vi "Ocelot.vi"(9 "RCW (X2)":dbl(slide) scale=-1.0..1.0, 10 "FWD (Y)":dbl(slide) scale=-1.0..1.0, 11 "STR (X)":dbl(slide) scale=-1.0..1.0) -> (0 "FRD":dbl(slide) scale=-1.0..1.0, 1 "FLD":dbl(slide) scale=-1.0..1.0, 2 "BRS":dbl(knob) scale=0.0..360.0, 3 "BLS":dbl(knob) scale=0.0..360.0, 4 "BLD":dbl(slide) scale=-1.0..1.0, 5 "FRS":dbl(knob) scale=0.0..360.0, 6 "BRD":dbl(slide) scale=-1.0..1.0, 7 "FLS":dbl(knob) scale=0.0..360.0)   [LabVIEW 2012]
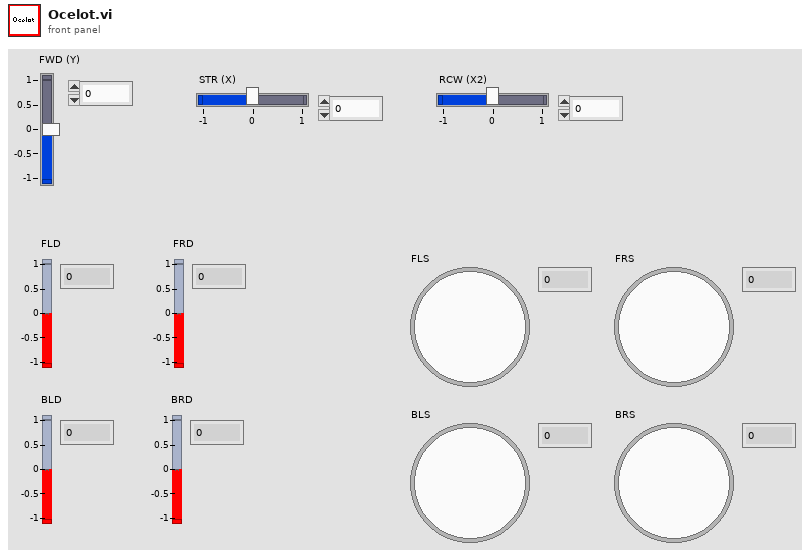
[diagram p1: front panel]
types:
  T1 = cluster{"WD1":dbl, "WD2":dbl, "WD3":dbl, "WD4":dbl}
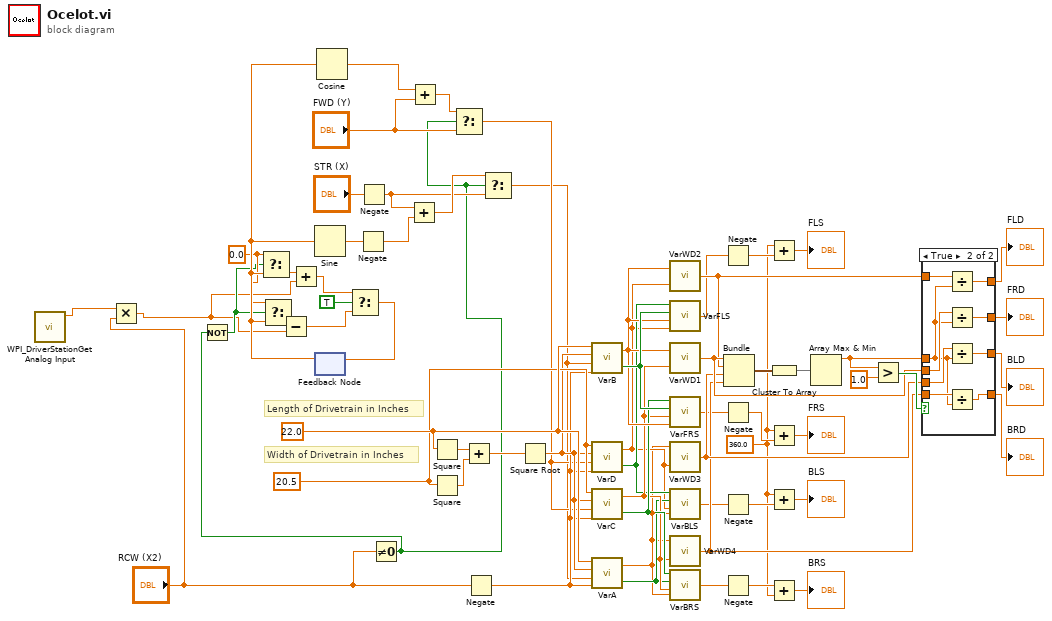
[diagram p0: block diagram]
diagram:
  w6 = 0.0 ("t")
  w32 = 360.0
  w59 = 20.5 ("W")
  w61 = 22.0 ("L")
  # "Length of Drivetrain in Inches"
  # "Width of Drivetrain in Inches"
  n1 = call <vilib>:"WPI_DriverStationGet Analog Input.vi"() -> ("Analog 1 (V)"=w1:dbl)  [unwired: 8 in, 3 out]
  n2 = Multiply(x=w1, y="RCW (X2)") -> (x*y=w2:dbl)
  n3 = feedback #1() -> (w19:dbl)  [unwired: 1 in]
  n4 = Sine(x=w19) -> (sin(x)=w14:dbl)
  n5 = Cosine(x=w19) -> (cos(x)=w18:dbl)
  n6 = Negate(x=w14) -> (-x=w13:dbl)
  n7 = Negate(x="STR (X)") -> (-x=w11:dbl)
  n8 = Not Equal To 0?(x="RCW (X2)") -> (x != 0?=w4:bool)
  n9 = Not(x=w4) -> (.not. x?=w5:bool)
  n10 = Select(t=w6, s=w5, f=w19) -> (s? t:f=w8:dbl)
  n11 = Select(t=w6, s=w5, f=w19) -> (s? t:f=w7:dbl)
  n12 = Subtract(x=w7, y=w2) -> (x-y=w22:dbl)
  n13 = Add(x=w8, y=w2) -> (x+y=w21:dbl)
  n14 = Select(t=w21, s=TRUE, f=w22) -> (s? t:f=w20:dbl)
  n15 = feedback-in #1(w20) -> ()
  n16 = Add(x=w11, y=w13) -> (x+y=w12:dbl)
  n17 = Add(x=w18, y="FWD (Y)") -> (x+y=w17:dbl)
  n18 = Square(x=w61) -> (x^2=w64:dbl)
  n19 = Square(x=w59) -> (x^2=w63:dbl)
  n20 = Select(t=w17, s=w4, f="FWD (Y)") -> (s? t:f=w16:dbl)
  n21 = Add(x=w64, y=w63) -> (x+y=w62:dbl)
  n22 = Negate(x="RCW (X2)") -> (-x=w23:dbl)
  n23 = Select(t=w12, s=w4, f=w11) -> (s? t:f=w10:dbl)
  n24 = Square Root(x=w62) -> (sqrt(x)=w58:dbl)
  n25 = call "VarB.vi"("RCW (X2)"=w23, "STR (X)"=w10, "R"=w58, "L"=w61) -> ("B = 0?"=w48:bool, "B"=w47:dbl)
  n26 = call "VarD.vi"("RCW (X2)"=w23, "FWD (Y)"=w16, "R"=w58, "W"=w59) -> ("x = 0?"=w44:bool, "D"=w42:dbl)
  n27 = call "VarC.vi"("RCW (X2)"=w23, "FWD (Y)"=w16, "R"=w58, "W"=w59) -> ("C = 0?"=w46:bool, "C"=w45:dbl)
  n28 = call "VarA.vi"("RCW (X2)"=w23, "STR (X)"=w10, "R"=w58, "L"=w61) -> ("A = 0?"=w43:bool, "A"=w41:dbl)
  n29 = call "VarWD2.vi"("D"=w42, "B"=w47) -> ("WD2"=w52:dbl)
  n30 = call "VarFLS.vi"("D"=w42, "B"=w47, "B=0"=w48, "D=0"=w44) -> ("FLS"=w25:dbl)
  n31 = call "VarWD1.vi"("C"=w45, "B"=w47) -> ("WD1"=w53:dbl)
  n32 = call "VarFRS.vi"("B"=w47, "C"=w45, "B=0"=w48, "C=0"=w46) -> ("FRS"=w27:dbl)
  n33 = call "VarWD3.vi"("D"=w42, "A"=w41) -> ("WD3"=w51:dbl)
  n34 = call "VarBLS.vi"("A"=w41, "D"=w42, "A=0"=w43, "D=0"=w44) -> ("BLS"=w29:dbl)
  n35 = call "VarWD4.vi"("C"=w45, "A"=w41) -> ("WD4"=w50:dbl)
  n36 = call "VarBRS.vi"("A"=w41, "C"=w45, "A=0"=w43, "C=0"=w46) -> ("BRS"=w31:dbl)
  n37 = Negate(x=w25) -> (-x=w36:dbl)
  n38 = Negate(x=w27) -> (-x=w35:dbl)
  n39 = Negate(x=w29) -> (-x=w34:dbl)
  n40 = Negate(x=w31) -> (-x=w33:dbl)
  n41 = Bundle("WD1"=w53, "WD2"=w52, "WD3"=w51, "WD4"=w50) -> (w56:T1)  [unwired: 1 in]
  n42 = Add(x=w32, y=w36) -> (x+y=→"FLS":dbl)
  n43 = Cluster To Array(cluster=w56) -> (array=w57:dbl[])
  n44 = Add(x=w32, y=w35) -> (x+y=→"FRS":dbl)
  n45 = Add(x=w32, y=w34) -> (x+y=→"BLS":dbl)
  n46 = Add(x=w33, y=w32) -> (x+y=→"BRS":dbl)
  n47 = Array Max & Min(array=w57) -> (max value=w49:dbl)  [unwired: 3 out]
  n48 = Greater?(x=w49, y=1.0) -> (0:w54:bool)
  n49 = case shown="True" w54 {
    tunnel: [w68 w73] -> w39
    tunnel: w53 -> [w68 w76]
    tunnel: w52 -> [w67 w77]
    tunnel: w51 -> [w66 w74]
    tunnel: w50 -> [w65 w75]
    tunnel: [w67 w72] -> w40
    tunnel: [w66 w71] -> w38
    tunnel: [w65 w69] -> w37
    tunnel: w49 -> [_ w70]
    frame False {
    }
    frame True {
      n50 = Divide(x=w77, y=w70) -> (x/y=w72:dbl)
      n51 = Divide(x=w76, y=w70) -> (x/y=w73:dbl)
      n52 = Divide(x=w74, y=w70) -> (x/y=w71:dbl)
      n53 = Divide(x=w75, y=w70) -> (x/y=w69:dbl)
    }
  }
  "FRD" <- w39
  "FLD" <- w40
  "BLD" <- w38
  "BRD" <- w37
